vi "Gyro Angle.vi"() -> ()   [LabVIEW 2014]
panel:
  out "Gyro Angle":dbl
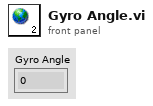
[diagram p1: front panel]
diagram:
